vi "Remove_selected_error.vi"(1 "error in (no error)":errorcluster, 2 "errorCode":i32) -> (0 "error out":errorcluster)   [LabVIEW 2014]
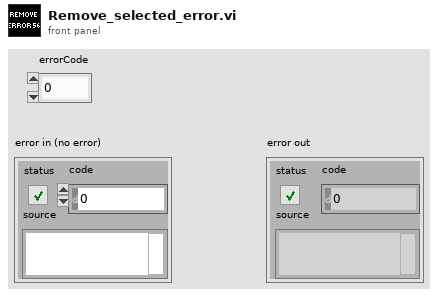
[diagram p1: front panel]
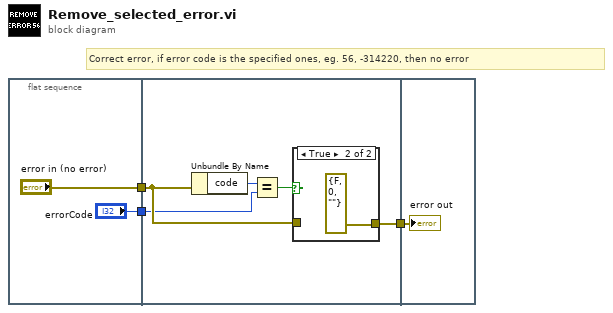
[diagram p0: block diagram]
diagram:
  # "Correct error, if error code is the specified ones, eg. 56, -314220, then no error"
  n1 = flat-sequence {
    tunnel: ["error in (no error)"] -> w3
    tunnel: ["errorCode"] -> w1
    tunnel: w3 -> [w8]
    tunnel: [w7] -> w2
    tunnel: w1 -> [w6]
    tunnel: w2 -> [w13]
    frame #0 {
    }
    frame #1 {
      n2 = Unbundle By Name(w8) -> ("code"=w10:i32)
      n3 = Equal?(x=w10, y=w6) -> (x = y?=w9:bool)
      n4 = case shown="True" w9 {
        tunnel: w8 -> [w11 _]
        tunnel: [w11 errorcluster {"status"=FALSE, "code"=0, "source"=""} ("error out")] -> w7
        frame False {
        }
        frame True {
        }
      }
    }
    frame #2 {
      "error out" <- w13
    }
  }
